vi "GetCurrentFileDirectory.vi"(8 "error in (no error)":errorcluster) -> (0 "error out":errorcluster, 3 "directory":path)   [LabVIEW 2017, in "FileManager.lvlib"]
uses:
  <vilib>/addons/InsightCM/Devices/Shared/Common/FileManager/FileManager.lvlib
  <vilib>/addons/InsightCM/Utilities/GlobalConfiguration/GlobalConfiguration.lvlib
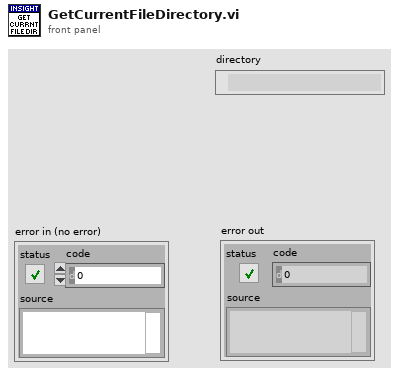
[diagram p1: front panel]
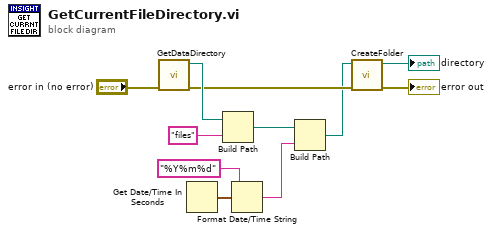
[diagram p0: block diagram]
diagram:
  n1 = call <vilib>:"GetDataDirectory.vi"("error in (no error)"="error in (no error)") -> ("error out"=w4:errorcluster, "data directory"=w10:path)  [unwired: 9 in]
  n2 = Get Date/Time In Seconds() -> (seconds since 1Jan1904=w8:timestamp)
  n3 = Build Path(base path=w10, name or relative path="files") -> (appended path=w6:path)
  n4 = Format Date/Time String(time format string (%c)="%Y%m%d", seconds (now)=w8) -> (date/time string=w5:string)  [unwired: 1 in]
  n5 = Build Path(base path=w6, name or relative path=w5) -> (appended path=w2:path)
  n6 = call <vilib>:"CreateFolder.vi"("error in (no error)"=w4, "folder"=w2) -> ("error out"=→"error out":errorcluster, "folder out"=→"directory":path)  [unwired: 8 in]
